vi "Set Rows Count.vi"(8 "error in":errorcluster, 10 "Rows Count":i32, 11 "SourceGrid in":refnum<class "SourceGrid.lvclass">) -> (0 "error out":errorcluster, 3 "SourceGrid out":refnum<class "SourceGrid.lvclass">)   [LabVIEW 2024, in "SourceGrid.lvlib" / "SourceGrid.lvclass"]
uses:
  SourceGrid.lvclass
  SourceGrid.lvclass/SourceGrid.ctl
  D:/git/Sourcegrid-LabVIEW/dll/SourceGrid.dll
  dll/SourceGrid.dll
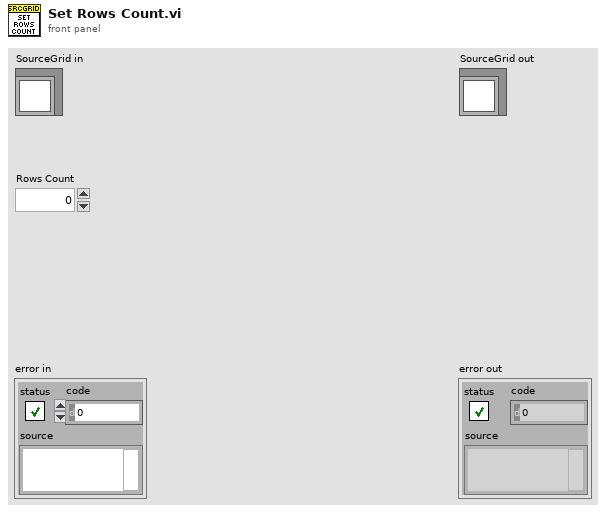
[diagram p1: front panel]
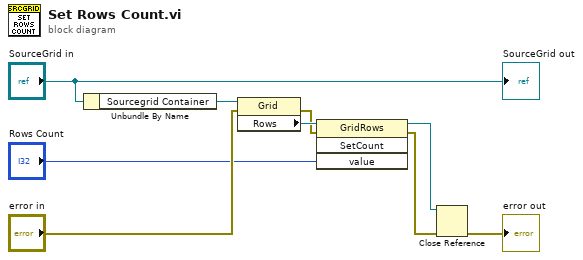
[diagram p0: block diagram]
diagram:
  n1 = Unbundle By Name("SourceGrid in") -> ("Sourcegrid Container"=w8:refnum<k24>)
  n2 = property class="Grid"(reference=w8, error in="error in") -> (error out=w6:errorcluster, "Rows"=w7:refnum<k24>)  [unwired: 1 out]
  n3 = invoke class="GridRows" method="SetCount"(reference=w7, error in=w6, "value"="Rows Count") -> (reference out=w1:refnum<k24>, error out=w3:errorcluster)  [unwired: 1 in, 2 out]
  n4 = Close Reference(reference=w1, error in (no error)=w3) -> (error out=→"error out":errorcluster)
  "SourceGrid out" <- "SourceGrid in"
